vi "testUIPanelCloseifpreviouslyclosed.vi"(8 "error in (no error)":errorcluster, 11 "testStateMachineUtilities in":refnum<class "testStateMachineUtilities.lvclass">) -> (0 "error out":errorcluster, 3 "testStateMachineUtilities out":refnum<class "testStateMachineUtilities.lvclass">)   [LabVIEW 2020, in "testStateMachineUtilities.lvclass"]
uses:
  testStateMachineUtilities.lvclass
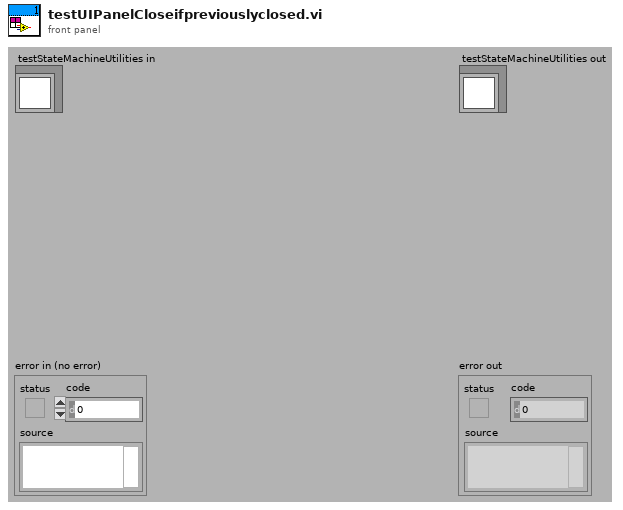
[diagram p1: front panel]
types:
  T1 = enum32{"Bad", "Idle", "Run top level", "Running"}
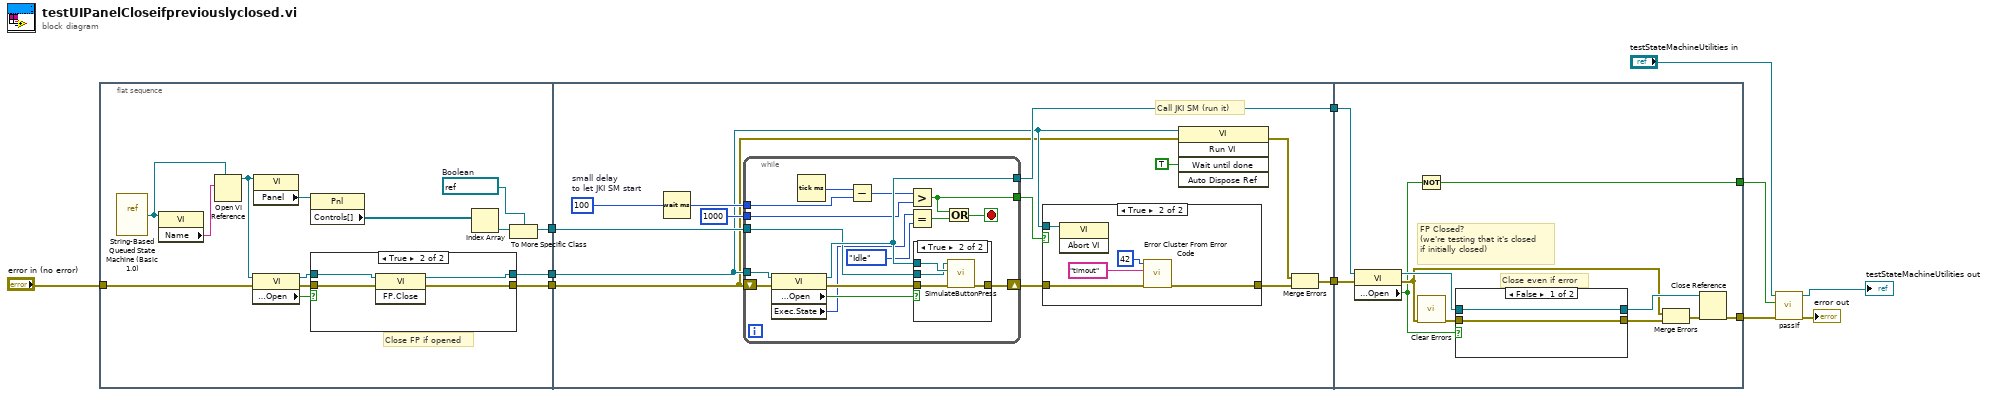
[diagram p0: block diagram]
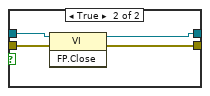
[diagram p5: hidden frame]
diagram:
  n1 = flat-sequence {
    tunnel: [w25] -> w11
    tunnel: [w24] -> w10
    tunnel: "error in (no error)" -> [w15]
    tunnel: [w19] -> w9
    tunnel: w11 -> [w36]
    tunnel: [w44] -> w8
    tunnel: [w33] -> w7
    tunnel: w10 -> [w34]
    tunnel: w9 -> [w43]
    tunnel: w8 -> [w82]
    tunnel: [w73] -> w6
    tunnel: [w77] -> w5
    tunnel: w7 -> [w81]
    frame #0 {
      w20 = refnum<vi> refnum  # Boolean
      # "Close FP if opened"
      n2 = vi-ref "String-Based Queued State Machine (Basic 1.0).vi"() -> (w17:refnum<vi>)
      n3 = property class="VI"(reference=w17) -> ("Name"=w18:string)  [unwired: 1 in, 2 out]
      n4 = Open VI Reference(type specifier VI Refnum (for type only)=w17, vi path=w18) -> (vi reference=w16:refnum<vi>)  [unwired: 4 in, 1 out]
      n5 = property class="VI"(reference=w16, error in=w15) -> (reference out=w14:refnum<vi>, error out=w13:errorcluster, "Front Panel.Open"=w12:bool)
      n6 = property class="VI"(reference=w16) -> ("Panel"=w23:refnum<vi>)  [unwired: 1 in, 2 out]
      n7 = property class="Pnl"(reference=w23) -> ("Controls[]"=w22:refnum<vi>[])  [unwired: 1 in, 2 out]
      n8 = case shown="True" w12 {
        tunnel: [w27 w29] -> w25
        tunnel: [w26 w28] -> w24
        tunnel: w14 -> [w27 w30]
        tunnel: w13 -> [w26 w31]
        frame False {
        }
        frame True {
          n9 = invoke class="VI" method="FP.Close"(reference=w30, error in=w31) -> (reference out=w29:refnum<vi>, error out=w28:errorcluster)  [unwired: 1 in, 1 out]
        }
      }
      n10 = Index Array(array=w22) -> (element=w21:refnum<vi>)  [unwired: 1 in]
      n11 = To More Specific Class(target class=w20, reference=w21) -> (specific class reference=w19:refnum<vi>)  [unwired: 1 in, 1 out]
    }
    frame #1 {
      w42 = u32 100  # small delay to let JKI SM start
      # "Call JKI SM (run it)"
      n12 = Wait (ms)(milliseconds to wait=w42) -> (millisecond timer value=w41:u32)
      n13 = while {
        tunnel: w36 -> [w66]
        tunnel: [w62] -> w44
        shift-right: [w65] -> w38
        shift-left: w34 -> [w64]
        tunnel: w43 -> [w61]
        tunnel: w41 -> [w59]
        tunnel: u32 1000 ("milliseconds to wait") -> [w57]
        tunnel: [w54] -> w39
        stop <- w55 stop-if-true
        n14 = property class="VI"(reference=w66, error in=w64) -> (reference out=w62:refnum<vi>, error out=w63:errorcluster, "Front Panel.Open"=w56:bool, "Exec.State"=w53:T1)
        n15 = Tick Count (ms)() -> (millisecond timer value=w60:u32)
        n16 = Subtract(x=w60, y=w59) -> (x-y=w58:u32)
        n17 = Greater?(x=w58, y=w57) -> (0:w54:bool)
        n18 = Equal?(x=w53, y=T1."Idle" ("Execution:State")) -> (x = y?=w51:bool)
        n19 = case shown="True" w56 {
          tunnel: [w67 w69] -> w65
          tunnel: w63 -> [w67 w68]
          tunnel: w62 -> [_ w71]
          tunnel: w61 -> [_ w70]
          frame False {
          }
          frame True {
            n20 = call "SimulateButtonPress.vi"("error in (no error)"=w68, "VIRef"=w71, "BooleanCtrlRef"=w70) -> ("error out"=w69:errorcluster)  [unwired: 8 in]
          }
        }
        n21 = Or(x=w54, y=w51) -> (x .or. y?=w55:bool)
      }
      n22 = case shown="True" w39 {
        tunnel: w36 -> [_ w50]
        tunnel: w38 -> [w45 w49]
        tunnel: [w45 w48] -> w37
        frame False {
        }
        frame True {
          n23 = invoke class="VI" method="Abort VI"(reference=w50) -> ()  [unwired: 2 in, 3 out]
          n24 = call <vilib>:"Error Cluster From Error Code.vi"("error in (no error)"=w49, "error message (\"\")"="timout" ("error message (\"\")"), "error code (0)"=42) -> ("error out"=w48:errorcluster)  [unwired: 6 in]
        }
      }
      n25 = invoke class="VI" method="Run VI"(reference=w36, error in=w34, "Wait until done"=TRUE ("Wait Until Done")) -> (error out=w32:errorcluster)  [unwired: 2 in, 4 out]
      n26 = Merge Errors(w32, w37) -> (w33:errorcluster)
    }
    frame #2 {
      # "FP Closed?\n(we're testing that it's closed\nif initially closed)"
      # "Close even if error"
      n27 = property class="VI"(reference=w82, error in=w81) -> (reference out=w80:refnum<vi>, error out=w75:errorcluster, "Front Panel.Open"=w72:bool)
      n28 = Not(x=w72) -> (.not. x?=w73:bool)
      n29 = call <vilib>:"Clear Errors.vi"("error in (no error)"=w75) -> ("error out"=w74:errorcluster)  [unwired: 5 in, 1 out]
      n30 = case shown="False" w72 {
        tunnel: w80 -> [w84 w88]
        tunnel: [w84 w87] -> w79
        tunnel: [w83 w86] -> w78
        tunnel: w74 -> [w83 w85]
        frame False {
        }
        frame True {
          n31 = invoke class="VI" method="FP.Close"(reference=w88, error in=w85) -> (reference out=w87:refnum<vi>, error out=w86:errorcluster)  [unwired: 1 in, 1 out]
        }
      }
      n32 = Merge Errors(w75, w78) -> (w76:errorcluster)
      n33 = Close Reference(reference=w79, error in (no error)=w76) -> (error out=w77:errorcluster)
    }
  }
  n34 = call-dynamic "passIf.vi"("error in (no error)"=w5, "pass"=w6, "TestCase in"="testStateMachineUtilities in") -> ("error out"=→"error out":errorcluster, "TestCase out"=→"testStateMachineUtilities out":refnum<class "testStateMachineUtilities.lvclass">)  [unwired: 7 in]
